vi "ReadIni.vi"(8 "Error In":errorcluster) -> (0 "Error Out":errorcluster, 3 "InternalData":T1)   [LabVIEW 2017, in "Client.lvlib" / "CommsFrameWork.lvlib"]
uses:
  CommsFrameWork.lvlib
  NI_LVConfig.lvlib
  Client.lvlib
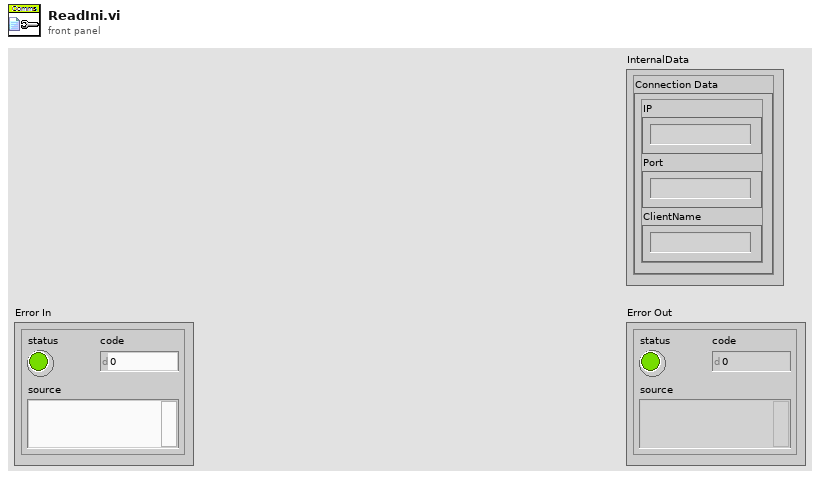
[diagram p1: front panel]
types:
  T1 = cluster{"Connection Data":cluster{"IP":string, "Port":string, "ClientName":string}}
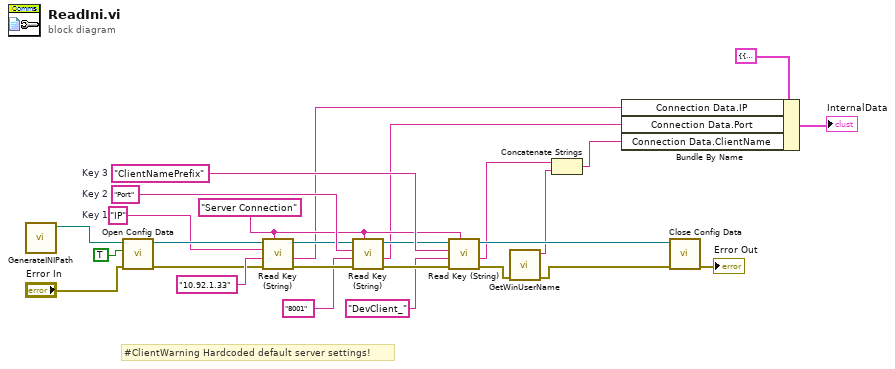
[diagram p0: block diagram]
diagram:
  w21 = "ClientNamePrefix"  # Key 3
  w20 = "Port"  # Key 2
  w19 = "IP"  # Key 1
  w18 = "Server Connection" ("section")
  # "#ClientWarning Hardcoded default server settings!"
  n1 = call "GenerateINIPath.vi"() -> ("INI Path"=w27:path)  [unwired: 11 in]
  n2 = call "Open Config Data.vi"("error in (no error)"="Error In", "create file if necessary (T)"=TRUE ("create file if necessary? (T)"), "configuration file path"=w27) -> ("error out"=w22:errorcluster, "refnum"=w23:refnum<k1>)  [unwired: 6 in, 1 out]
  n3 = call "Read Key (String).vi"("section"=w18, "error in (no error)"=w22, "default value"="10.92.1.33", "key"=w19, "refnum"=w23) -> ("error out"=w14:errorcluster, "value"=w12:string, "refnum out"=w15:refnum<k1>)  [unwired: 3 in, 1 out]
  n4 = call "Read Key (String).vi"("section"=w18, "error in (no error)"=w14, "default value"="8001", "key"=w20, "refnum"=w15) -> ("error out"=w17:errorcluster, "value"=w11:string, "refnum out"=w16:refnum<k1>)  [unwired: 3 in, 1 out]
  n5 = call "Read Key (String).vi"("section"=w18, "error in (no error)"=w17, "default value"="DevClient_", "key"=w21, "refnum"=w16) -> ("error out"=w4:errorcluster, "value"=w5:string, "refnum out"=w25:refnum<k1>)  [unwired: 3 in, 1 out]
  n6 = call "GetWinUserName.vi"("Error In"=w4) -> ("Error Out"=w3:errorcluster, "Windows User Name"=w7:string)  [unwired: 9 in]
  n7 = Concatenate Strings(w5, w7) -> (w6:string)
  n8 = Bundle By Name(cluster=T1 {"Connection Data"={"IP"="", "Port"="", "ClientName"=""}} ("InternalData"), "Connection Data.IP"=w12, "Connection Data.Port"=w11, "Connection Data.ClientName"=w6) -> (→"InternalData":T1)
  n9 = call "Close Config Data.vi"("error in (no error)"=w3, "refnum"=w25) -> ("error out"=→"Error Out":errorcluster)  [unwired: 1 in, 8 out]
